vi "Merge.vi"(10 "Cache Managers":refnum<class "ConfigManager.Cache.lvclass">[](array[class])) -> (2 "Merged Cache":refnum<class "ConfigManager.Cache.lvclass">)   [LabVIEW 2013, in "CfgManager.lvlib" / "ConfigManager.Cache.lvclass"]
uses:
  ConfigManager.Cache.lvclass
  ConfigManager.Cache.lvclass/ConfigManager.Cache.ctl
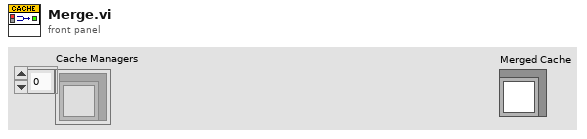
[diagram p1: front panel]
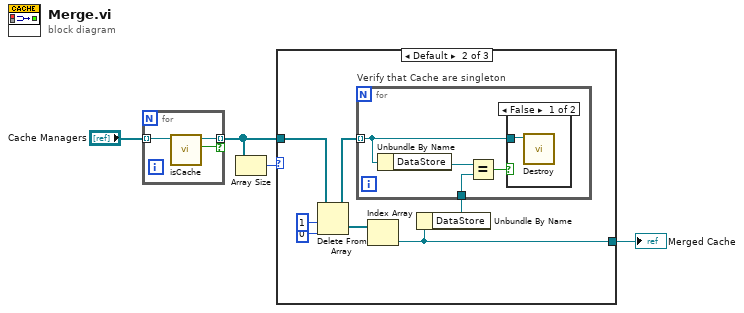
[diagram p0: block diagram]
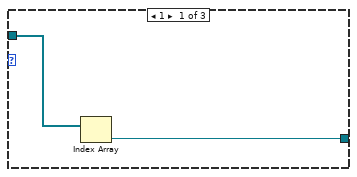
[diagram p2: hidden frame]
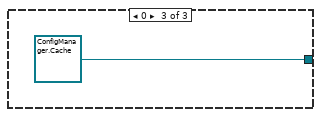
[diagram p4: hidden frame]
diagram:
  n1 = for {
    tunnel: "Cache Managers" -> [w7] mode=indexing
    tunnel: [w6] -> w3 mode=indexing if=w5
    n2 = call "isCache.vi"("ConfigManager.Cache in"=w7) -> ("isCache?"=w5:bool, "ConfigManager.Cache out"=w6:refnum<class "ConfigManager.Cache.lvclass">)  [unwired: 9 in]
  }
  n3 = Array Size(array=w3) -> (size(s)=w4:i32)
  n4 = case shown="1" w4 {
    tunnel: w3 -> [w9 w16 _]
    tunnel: [w8 w11 refnum<class "ConfigManager.Cache.lvclass"> refnum ("Cache")] -> w1
    frame 1 {
      n5 = Index Array(array=w9) -> (element=w8:refnum<class "ConfigManager.Cache.lvclass">)  [unwired: 1 in]
    }
    frame Default {
      n6 = Delete From Array(array=w16, length=1, index=0) -> (deleted portion=w13:refnum<class "ConfigManager.Cache.lvclass">[], array with subset deleted=w12:refnum<class "ConfigManager.Cache.lvclass">[])
      n7 = Index Array(array=w13) -> (element=w11:refnum<class "ConfigManager.Cache.lvclass">)  [unwired: 1 in]
      n8 = Unbundle By Name(w11) -> ("DataStore"=w10:refnum<data-value>)
      n9 = for "Verify that Cache are singleton" {
        tunnel: w12 -> [w17] mode=indexing
        tunnel: w10 -> [w19]
        n10 = Unbundle By Name(w17) -> ("DataStore"=w20:refnum<data-value>)
        n11 = Equal?(x=w20, y=w19) -> (x = y?=w18:bool)
        n12 = case shown="False" w18 {
          tunnel: w17 -> [w21 _]
          frame False {
            n13 = call-dynamic "Destroy.vi"("ConfigManager.Cache in"=w21) -> ()  [unwired: 9 in, 2 out]
          }
          frame True {
          }
        }
      }
    }
    frame 0 {
    }
  }
  "Merged Cache" <- w1
